vi "Host_StreamLoop.vi"(8 "error in (no error)":errorcluster) -> (0 "error out":errorcluster)   [LabVIEW 2018]
doc: "Loop containing the network stream for verifying connectivity with the target cRIO. Network stream is contained within a state machine that has initialization, read/write, wait, and terminate states. If for any reason the writer or the reader loops are stopped, the control on the front panel of Host__Main.vi \"Reinitialize Streams\" may be pressed to reconnect the streams. \nAlso contains the network shared variables that send data and actuations from the target cRIO and writes it to single-process variables on the host. Also collects the data in a shift register to be sent to the data logging vi, Host_SaveToFile.vi"
uses:
  Libraries/TypeDef_NetworkStreamState.ctl
  Master/Control/TypeDef_DigitalOuts.ctl
  Master/DAQ/Master_DataControl.ctl
  Master/DAQ/TypeDef_cRIOData.ctl
  Master/IMU/TypeDef_IMUData.ctl
  Master/CAN/TypeDef_BMSData.ctl
  Master/CAN/TypeDef_BMS_Status.ctl
  Master/CAN/MotorController/fixedMotorData.ctl
  Master/CAN/MotorController/MotorStatus.ctl
  Globals/Host_STOP.vi
  Globals/Host_DATAALL.vi
  <resource>/objmgr/ni.dex.rc
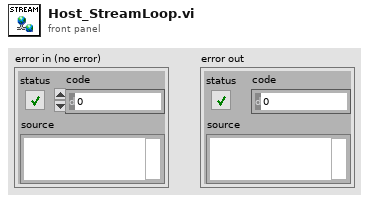
[diagram p1: front panel]
types:
  T1 = enum16{"Time", "24V Battery Voltage", "24V Battery Current", "Stripe Count", "Pressure Vessel Pressure", "Flow Sensor", "Fairing Temperature", "Reservoir Temperature", "RIght Hall Effect", "Left Hall Effect", "Tank Pressure", "Right Clamp Pressure", "Left Clamp Pressure", "Brake Pressure", "Cooling Pressure", "DIsplacement", "Velocity", "Acceleration", "Ambient Pressure", "IMU Temperature"}
  T2 = typedef "TypeDef_NetworkStreamState.ctl" = enum16{"Wait", "Test", "Initialize", "Read/Write", "Terminate"}
  T3 = typedef "TypeDef_DigitalOuts.ctl" = cluster{"Pod Power":bool, "Dump Valve":bool, "Brakes":bool, "Clamp":bool, "Pump":bool, "Ignition":bool, "DO6":bool, "DO7":bool, "HighSide":bool, "Precharge":bool, "LowSide":bool, "DO3":bool, "DO4":bool, "DO5":bool, "DO62":bool, "DO72":bool}
  T4 = typedef "Master_DataControl.ctl" = cluster{"cRIO Data":T5, "IMU Data":T6, "BMS Data":T7, "Motor Data":T9}
  T5 = typedef "TypeDef_cRIOData.ctl" = cluster{"Time (ms)":dbl, "24V Battery (V)":dbl, "LowV Current (A)":dbl, "Fiducial Sensor (V)":dbl, "PV Pressure (psig)":dbl, "Flow Sensor (V)":dbl, "Temp Fairing (F)":dbl, "Temp Reservoir (F)":dbl, "HallEffect Right (in)":dbl, "HallEffect Left (in)":dbl, "PT Tank (psig)":dbl, "PT Clamp Right (psig)":dbl, "PT Clamp Left (psig)":dbl, "PT Brake (psig)":dbl, "PT Cooling (psig)":dbl, "Displacement (ft)":dbl, "Velocity (ft/s)":dbl}
  T6 = typedef "TypeDef_IMUData.ctl" = cluster{"x acceleration (g)":dbl, "Pressure (psia)":dbl, "Temperature (F)":dbl}
  T7 = typedef "TypeDef_BMSData.ctl" = cluster{"Max Cell Voltage (V)":dbl, "Max Cell ID":dbl, "Min Cell Voltage (V)":dbl, "Min Cell ID":dbl, "State of Charge (%)":dbl, "Average Voltage (V)":dbl, "Voltage Delta (V)":dbl, "Pack Current (A)":dbl, "Pack Voltage (V)":dbl, "Max Resistance (Ohm)":dbl, "Min Resistance (Ohm)":dbl, "Average Resistance (Ohm)":dbl, "Delta Resistance (Ohm)":dbl, "Highest Temperature(F)":dbl, "BmsStatus":T8}
  T8 = typedef "TypeDef_BMS_Status.ctl" = cluster{"isFault":bool, "isolationMonitoring":bool}
  T9 = typedef "fixedMotorData.ctl" = cluster{"Velo (RPM)":dbl, "MotorTemp(F)":dbl, "CtrlTemp(F)":dbl, "DcLinkVolt(V)":dbl, "ErrorCode":dbl, "motorStatus":T10, "isAlive":bool, "motorControllerState":u16}
  T10 = typedef "MotorStatus.ctl" = cluster{"isReady":bool, "isOn":bool, "isOperEn":bool, "isFault":bool, "isVoltEn":bool, "targetReached":bool, "isWarning":bool}
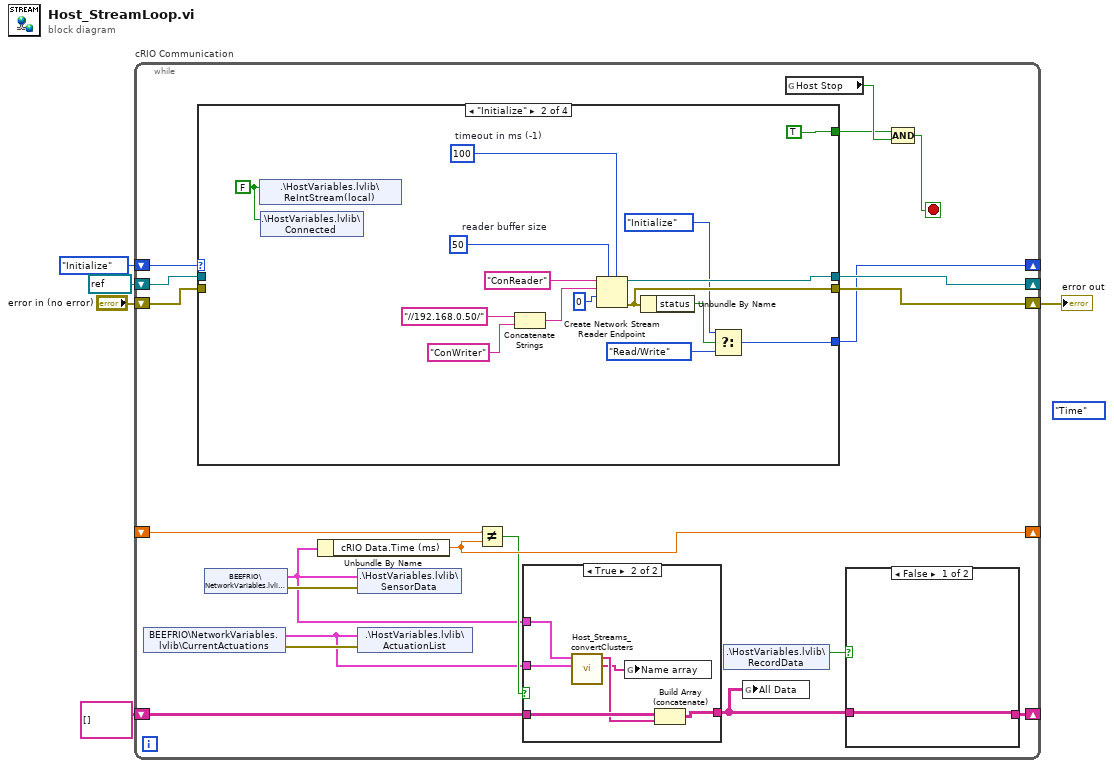
[diagram p0: block diagram]
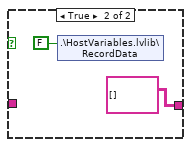
[diagram p2: hidden frame]
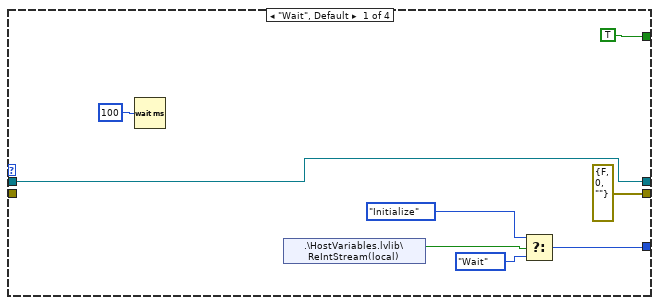
[diagram p4: hidden frame]
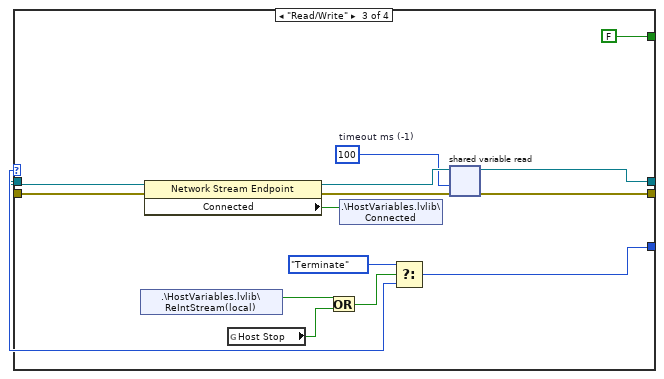
[diagram p5: hidden frame]
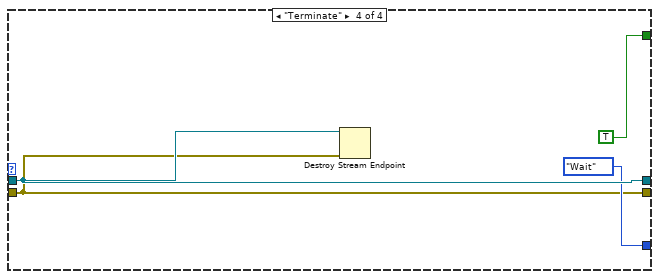
[diagram p6: hidden frame]
diagram:
  (unwired) T1."Time"
  n1 = while "cRIO Communication" {
    shift-right: [w20] -> w3
    shift-left: "error in (no error)" -> [w22]
    shift-right: [w21] -> _
    shift-left: refnum<k21> refnum ("reader name") -> [w23]
    shift-right: [w19] -> _
    shift-left: TypeDef_NetworkStreamState."Initialize" ("Enum out") -> [w18]
    shift-right: [w14] -> _
    shift-left: _ -> [w13]
    shift-right: [w10] -> _
    shift-left: string[][] [] -> [w7]
    stop <- w25 stop-if-true
    n2 = shared-variable "BEEFRIO\\NetworkVariables.lvlib\\CurrentActuations"() -> (w11:T3, error out=w16:errorcluster)  [unwired: 1 in]
    n3 = case shown="\"Initialize\"" w18 {
      selector: w18 -> [_ _ w73 _]
      tunnel: [w43 w58 w65 w77] -> w21
      tunnel: [errorcluster {"status"=FALSE, "code"=0, "source"=""} ("error IO") w57 w63 w75] -> w20
      tunnel: w22 -> [_ _ w68 w75]
      tunnel: w23 -> [w43 _ w69 w77]
      tunnel: [w39 w53 w72 TypeDef_NetworkStreamState."Wait"] -> w19
      tunnel: [TRUE TRUE FALSE TRUE] -> w17
      frame "Wait", Default {
        n4 = Wait (ms)(milliseconds to wait=u32 100) -> ()  [unwired: 1 out]
        n5 = shared-variable ".\\HostVariables.lvlib\\ReIntStream(local)"() -> (w36:bool)  [unwired: 1 in, 1 out]
        n6 = Select(t=TypeDef_NetworkStreamState."Initialize", s=w36, f=TypeDef_NetworkStreamState."Wait") -> (s? t:f=w39:T2)
      }
      frame "Initialize" {
        w44 = FALSE ("ReIntStream(local)")
        w48 = 100  # timeout in ms (-1)
        w49 = 50  # reader buffer size
        n7 = shared-variable ".\\HostVariables.lvlib\\ReIntStream(local)"(w44) -> ()  [unwired: 1 in, 1 out]
        n8 = shared-variable ".\\HostVariables.lvlib\\Connected"(w44) -> ()  [unwired: 1 in, 1 out]
        n9 = Concatenate Strings("//192.168.0.50/", "ConWriter" ("reader url")) -> (w46:string)
        n10 = Create Network Stream Reader Endpoint(5:w48, 7:w49, 9:i8 0, 10:w46, 11:"ConReader" ("reader name")) -> (0:w57:errorcluster, 3:w58:refnum<k21>)  [unwired: 2 in]
        n11 = Unbundle By Name(w57) -> ("status"=w56:bool)
        n12 = Select(t=TypeDef_NetworkStreamState."Initialize" ("Enum"), s=w56, f=TypeDef_NetworkStreamState."Read/Write" ("Enum")) -> (s? t:f=w53:T2)
      }
      frame "Read/Write" {
        w62 = 100  # timeout ms (-1)
        n13 = shared-variable ".\\HostVariables.lvlib\\ReIntStream(local)"() -> (w59:bool)  [unwired: 1 in, 1 out]
        n14 = property class="Network Stream Endpoint"(reference=w69, error in=w68) -> (reference out=w66:refnum<k21>, error out=w64:errorcluster, "Connected"=w61:bool)
        n15 = global read "Host_STOP.vi" "Host Stop"() -> (w67:bool)
        n16 = Or(x=w59, y=w67) -> (x .or. y?=w60:bool)
        n17 = shared-variable ".\\HostVariables.lvlib\\Connected"(w61) -> ()  [unwired: 1 in, 1 out]
        n18 = Select(t=TypeDef_NetworkStreamState."Terminate", s=w60, f=w73) -> (s? t:f=w72:T2)
        n19 = shared-variable-read(w66, w64, w62) -> (w65:refnum<k21>, w63:errorcluster)  [unwired: 2 out]
      }
      frame "Terminate" {
        n20 = Destroy Stream Endpoint(8:w75, 11:w77) -> ()  [unwired: 1 out]
      }
    }
    n21 = shared-variable "BEEFRIO\\NetworkVariables.lvlib\\AllData"() -> (w6:T4, error out=w15:errorcluster)  [unwired: 1 in]
    n22 = Unbundle By Name(w6) -> ("cRIO Data.Time (ms)"=w14:dbl)
    n23 = shared-variable ".\\HostVariables.lvlib\\SensorData"(w6, error in=w15) -> ()  [unwired: 1 out]
    n24 = shared-variable ".\\HostVariables.lvlib\\ActuationList"(w11, error in=w16) -> ()  [unwired: 1 out]
    n25 = Not Equal?(x=w13, y=w14) -> (x != y?=w12:bool)
    n26 = case shown="True" w12 {
      tunnel: [w29 w35] -> w8
      tunnel: w7 -> [w29 w34]
      tunnel: w6 -> [_ w33]
      tunnel: w11 -> [_ w32]
      frame False {
      }
      frame True {
        n27 = call "Host_Streams_convertClusters.vi"("Actuators in"=w32, "Data in"=w33) -> ("Name array"=w30:string[], "Info array"=w31:string[])  [unwired: 8 in]
        n28 = global write "Host_DATAALL.vi" "Name array"(w30) -> ()
        n29 = Build Array (concatenate)(w34, w31) -> (w35:string[][])
      }
    }
    n30 = shared-variable ".\\HostVariables.lvlib\\RecordData"() -> (w9:bool)  [unwired: 1 in, 1 out]
    n31 = global write "Host_DATAALL.vi" "All Data"(w8) -> ()
    n32 = global read "Host_STOP.vi" "Host Stop"() -> (w24:bool)
    n33 = case shown="False" w9 {
      tunnel: w8 -> [w26 _]
      tunnel: [w26 string[][] []] -> w10
      frame False {
      }
      frame True {
        n34 = shared-variable ".\\HostVariables.lvlib\\RecordData"(FALSE ("RecordData")) -> ()  [unwired: 1 in, 1 out]
      }
    }
    n35 = Compound Arithmetic op=AND(w17, w24) -> (w25:bool)
  }
  "error out" <- w3
